vi "App - analyze RUS V6.vi"() -> ()   [LabVIEW 2015] (continued)
"last mod"=timestamp(3493785599 s since 1904-01-01), "file name str"="D:\\Data\\Ultrasound\\LSCO\\LSCO22__130814c\\5_Cooling_2nd_try\\September_2014\\091714\\72.10600K_500_2500_2.10000V_0.00000T_Sep17-2014__03-59-59_001_091714.bin", "mod time(min)"=58229759.983333334, "file format"=enum."binary", "power(V)"=2.1, "Magn Field(T) "=0.0}, {"temperature"=72.039, "temperature str"="72.03900", "file path"=path "D:/Data/Ultrasound/LSCO/LSCO22__130814c/5_Cooling_2nd_try/September_2014/091714/72.03900K_500_2500_2.10000V_0.00000T_Sep17-2014__04-01-18_001_091714.bin", "last mod"=timestamp(3493785678 s since 1904-01-01), "file name str"="D:\\Data\\Ultrasound\\LSCO\\LSCO22__130814c\\5_Cooling_2nd_try\\September_2014\\091714\\72.03900K_500_2500_2.10000V_0.00000T_Sep17-2014__04-01-18_001_091714.bin", "mod time(min)"=58229761.3, "file format"=enum."binary", "power(V)"=2.1, "Magn Field(T) "=0.0}, {"temperature"=71.974, "temperature str"="71.97400", "file path"=path "D:/Data/Ultrasound/LSCO/LSCO22__130814c/5_Cooling_2nd_try/September_2014/091714/71.97400K_500_2500_2.10000V_0.00000T_Sep17-2014__04-02-38_001_091714.bin", "last mod"=timestamp(3493785758 s since 1904-01-01), "file name str"="D:\\Data\\Ultrasound\\LSCO\\LSCO22__130814c\\5_Cooling_2nd_try\\September_2014\\091714\\71.97400K_500_2500_2.10000V_0.00000T_Sep17-2014__04-02-38_001_091714.bin", "mod time(min)"=58229762.63333333, "file format"=enum."binary", "power(V)"=2.1, "Magn Field(T) "=0.0}, {"temperature"=71.908, "temperature str"="71.90800", "file path"=path "D:/Data/Ultrasound/LSCO/LSCO22__130814c/5_Cooling_2nd_try/September_2014/091714/71.90800K_500_2500_2.10000V_0.00000T_Sep17-2014__04-03-57_001_091714.bin", "last mod"=timestamp(3493785837 s since 1904-01-01), "file name str"="D:\\Data\\Ultrasound\\LSCO\\LSCO22__130814c\\5_Cooling_2nd_try\\September_2014\\091714\\71.90800K_500_2500_2.10000V_0.00000T_Sep17-2014__04-03-57_001_091714.bin", "mod time(min)"=58229763.95, "file format"=enum."binary", "power(V)"=2.1, "Magn Field(T) "=0.0}, {"temperature"=71.842, "temperature str"="71.84200", "file path"=path "D:/Data/Ultrasound/LSCO/LSCO22__130814c/5_Cooling_2nd_try/September_2014/091714/71.84200K_500_2500_2.10000V_0.00000T_Sep17-2014__04-05-17_001_091714.bin", "last mod"=timestamp(3493785917 s since 1904-01-01), "file name str"="D:\\Data\\Ultrasound\\LSCO\\LSCO22__130814c\\5_Cooling_2nd_try\\September_2014\\091714\\71.84200K_500_2500_2.10000V_0.00000T_Sep17-2014__04-05-17_001_091714.bin", "mod time(min)"=58229765.28333333, "file format"=enum."binary", "power(V)"=2.1, "Magn Field(T) "=0.0}, {"temperature"=71.776, "temperature str"="71.77600", "file path"=path "D:/Data/Ultrasound/LSCO/LSCO22__130814c/5_Cooling_2nd_try/September_2014/091714/71.77600K_500_2500_2.10000V_0.00000T_Sep17-2014__04-06-36_001_091714.bin", "last mod"=timestamp(3493785996 s since 1904-01-01), "file name str"="D:\\Data\\Ultrasound\\LSCO\\LSCO22__130814c\\5_Cooling_2nd_try\\September_2014\\091714\\71.77600K_500_2500_2.10000V_0.00000T_Sep17-2014__04-06-36_001_091714.bin", "mod time(min)"=58229766.6, "file format"=enum."binary", "power(V)"=2.1, "Magn Field(T) "=0.0}, {"temperature"=71.708, "temperature str"="71.70800", "file path"=path "D:/Data/Ultrasound/LSCO/LSCO22__130814c/5_Cooling_2nd_try/September_2014/091714/71.70800K_500_2500_2.10000V_0.00000T_Sep17-2014__04-07-55_001_091714.bin", "last mod"=timestamp(3493786075 s since 1904-01-01), "file name str"="D:\\Data\\Ultrasound\\LSCO\\LSCO22__130814c\\5_Cooling_2nd_try\\September_2014\\091714\\71.70800K_500_2500_2.10000V_0.00000T_Sep17-2014__04-07-55_001_091714.bin", "mod time(min)"=58229767.916666664, "file format"=enum."binary", "power(V)"=2.1, "Magn Field(T) "=0.0}, {"temperature"=71.643, "temperature str"="71.64300", "file path"=path "D:/Data/Ultrasound/LSCO/LSCO22__130814c/5_Cooling_2nd_try/September_2014/091714/71.64300K_500_2500_2.10000V_0.00000T_Sep17-2014__04-09-15_001_091714.bin", "last mod"=timestamp(3493786155 s since 1904-01-01), "file name str"="D:\\Data\\Ultrasound\\LSCO\\LSCO22__130814c\\5_Cooling_2nd_try\\September_2014\\091714\\71.64300K_500_2500_2.10000V_0.00000T_Sep17-2014__04-09-15_001_091714.bin", "mod time(min)"=58229769.25, "file format"=enum."binary", "power(V)"=2.1, "Magn Field(T) "=0.0}, {"temperature"=71.578, "temperature str"="71.57800", "file path"=path "D:/Data/Ultrasound/LSCO/LSCO22__130814c/5_Cooling_2nd_try/September_2014/091714/71.57800K_500_2500_2.10000V_0.00000T_Sep17-2014__04-10-34_001_091714.bin", "last mod"=timestamp(3493786234 s since 1904-01-01), "file name str"="D:\\Data\\Ultrasound\\LSCO\\LSCO22__130814c\\5_Cooling_2nd_try\\September_2014\\091714\\71.57800K_500_2500_2.10000V_0.00000T_Sep17-2014__04-10-34_001_091714.bin", "mod time(min)"=58229770.56666667, "file format"=enum."binary", "power(V)"=2.1, "Magn Field(T) "=0.0}, {"temperature"=71.514, "temperature str"="71.51400", "file path"=path "D:/Data/Ultrasound/LSCO/LSCO22__130814c/5_Cooling_2nd_try/September_2014/091714/71.51400K_500_2500_2.10000V_0.00000T_Sep17-2014__04-11-54_001_091714.bin", "last mod"=timestamp(3493786314 s since 1904-01-01), "file name str"="D:\\Data\\Ultrasound\\LSCO\\LSCO22__130814c\\5_Cooling_2nd_try\\September_2014\\091714\\71.51400K_500_2500_2.10000V_0.00000T_Sep17-2014__04-11-54_001_091714.bin", "mod time(min)"=58229771.9, "file format"=enum."binary", "power(V)"=2.1, "Magn Field(T) "=0.0}, {"temperature"=71.446, "temperature str"="71.44600", "file path"=path "D:/Data/Ultrasound/LSCO/LSCO22__130814c/5_Cooling_2nd_try/September_2014/091714/71.44600K_500_2500_2.10000V_0.00000T_Sep17-2014__04-13-13_001_091714.bin", "last mod"=timestamp(3493786393 s since 1904-01-01), "file name str"="D:\\Data\\Ultrasound\\LSCO\\LSCO22__130814c\\5_Cooling_2nd_try\\September_2014\\091714\\71.44600K_500_2500_2.10000V_0.00000T_Sep17-2014__04-13-13_001_091714.bin", "mod time(min)"=58229773.21666667, "file format"=enum."binary", "power(V)"=2.1, "Magn Field(T) "=0.0}, {"temperature"=71.383, "temperature str"="71.38300", "file path"=path "D:/Data/Ultrasound/LSCO/LSCO22__130814c/5_Cooling_2nd_try/September_2014/091714/71.38300K_500_2500_2.10000V_0.00000T_Sep17-2014__04-14-32_001_091714.bin", "last mod"=timestamp(3493786472 s since 1904-01-01), "file name str"="D:\\Data\\Ultrasound\\LSCO\\LSCO22__130814c\\5_Cooling_2nd_try\\September_2014\\091714\\71.38300K_500_2500_2.10000V_0.00000T_Sep17-2014__04-14-32_001_091714.bin", "mod time(min)"=58229774.53333333, "file format"=enum."binary", "power(V)"=2.1, "Magn Field(T) "=0.0}, {"temperature"=71.316, "temperature str"="71.31600", "file path"=path "D:/Data/Ultrasound/LSCO/LSCO22__130814c/5_Cooling_2nd_try/September_2014/091714/71.31600K_500_2500_2.10000V_0.00000T_Sep17-2014__04-15-52_001_091714.bin", "last mod"=timestamp(3493786552 s since 1904-01-01), "file name str"="D:\\Data\\Ultrasound\\LSCO\\LSCO22__130814c\\5_Cooling_2nd_try\\September_2014\\091714\\71.31600K_500_2500_2.10000V_0.00000T_Sep17-2014__04-15-52_001_091714.bin", "mod time(min)"=58229775.86666667, "file format"=enum."binary", "power(V)"=2.1, "Magn Field(T) "=0.0}, {"temperature"=71.25, "temperature str"="71.25000", "file path"=path "D:/Data/Ultrasound/LSCO/LSCO22__130814c/5_Cooling_2nd_try/September_2014/091714/71.25000K_500_2500_2.10000V_0.00000T_Sep17-2014__04-17-11_001_091714.bin", "last mod"=timestamp(3493786631 s since 1904-01-01), "file name str"="D:\\Data\\Ultrasound\\LSCO\\LSCO22__130814c\\5_Cooling_2nd_try\\September_2014\\091714\\71.25000K_500_2500_2.10000V_0.00000T_Sep17-2014__04-17-11_001_091714.bin", "mod time(min)"=58229777.18333333, "file format"=enum."binary", "power(V)"=2.1, "Magn Field(T) "=0.0}, {"temperature"=71.184, "temperature str"="71.18400", "file path"=path "D:/Data/Ultrasound/LSCO/LSCO22__130814c/5_Cooling_2nd_try/September_2014/091714/71.18400K_500_2500_2.10000V_0.00000T_Sep17-2014__04-18-30_001_091714.bin", "last mod"=timestamp(3493786710 s since 1904-01-01), "file name str"="D:\\Data\\Ultrasound\\LSCO\\LSCO22__130814c\\5_Cooling_2nd_try\\September_2014\\091714\\71.18400K_500_2500_2.10000V_0.00000T_Sep17-2014__04-18-30_001_091714.bin", "mod time(min)"=58229778.5, "file format"=enum."binary", "power(V)"=2.1, "Magn Field(T) "=0.0}, {"temperature"=71.122, "temperature str"="71.12200", "file path"=path "D:/Data/Ultrasound/LSCO/LSCO22__130814c/5_Cooling_2nd_try/September_2014/091714/71.12200K_500_2500_2.10000V_0.00000T_Sep17-2014__04-19-50_001_091714.bin", "last mod"=timestamp(3493786790 s since 1904-01-01), "file name str"="D:\\Data\\Ultrasound\\LSCO\\LSCO22__130814c\\5_Cooling_2nd_try\\September_2014\\091714\\71.12200K_500_2500_2.10000V_0.00000T_Sep17-2014__04-19-50_001_091714.bin", "mod time(min)"=58229779.833333336, "file format"=enum."binary", "power(V)"=2.1, "Magn Field(T) "=0.0}, {"temperature"=71.056, "temperature str"="71.05600", "file path"=path "D:/Data/Ultrasound/LSCO/LSCO22__130814c/5_Cooling_2nd_try/September_2014/091714/71.05600K_500_2500_2.10000V_0.00000T_Sep17-2014__04-21-09_001_091714.bin", "last mod"=timestamp(3493786869 s since 1904-01-01), "file name str"="D:\\Data\\Ultrasound\\LSCO\\LSCO22__130814c\\5_Cooling_2nd_try\\September_2014\\091714\\71.05600K_500_2500_2.10000V_0.00000T_Sep17-2014__04-21-09_001_091714.bin", "mod time(min)"=58229781.15, "file format"=enum."binary", "power(V)"=2.1, "Magn Field(T) "=0.0}, {"temperature"=70.993, "temperature str"="70.99300", "file path"=path "D:/Data/Ultrasound/LSCO/LSCO22__130814c/5_Cooling_2nd_try/September_2014/091714/70.99300K_500_2500_2.10000V_0.00000T_Sep17-2014__04-22-29_001_091714.bin", "last mod"=timestamp(3493786949 s since 1904-01-01), "file name str"="D:\\Data\\Ultrasound\\LSCO\\LSCO22__130814c\\5_Cooling_2nd_try\\September_2014\\091714\\70.99300K_500_2500_2.10000V_0.00000T_Sep17-2014__04-22-29_001_091714.bin", "mod time(min)"=58229782.483333334, "file format"=enum."binary", "power(V)"=2.1, "Magn Field(T) "=0.0}, {"temperature"=70.928, "temperature str"="70.92800", "file path"=path "D:/Data/Ultrasound/LSCO/LSCO22__130814c/5_Cooling_2nd_try/September_2014/091714/70.92800K_500_2500_2.10000V_0.00000T_Sep17-2014__04-23-48_001_091714.bin", "last mod"=timestamp(3493787028 s since 1904-01-01), "file name str"="D:\\Data\\Ultrasound\\LSCO\\LSCO22__130814c\\5_Cooling_2nd_try\\September_2014\\091714\\70.92800K_500_2500_2.10000V_0.00000T_Sep17-2014__04-23-48_001_091714.bin", "mod time(min)"=58229783.8, "file format"=enum."binary", "power(V)"=2.1, "Magn Field(T) "=0.0}, {"temperature"=70.86, "temperature str"="70.86000", "file path"=path "D:/Data/Ultrasound/LSCO/LSCO22__130814c/5_Cooling_2nd_try/September_2014/091714/70.86000K_500_2500_2.10000V_0.00000T_Sep17-2014__04-25-07_001_091714.bin", "last mod"=timestamp(3493787107 s since 1904-01-01), "file name str"="D:\\Data\\Ultrasound\\LSCO\\LSCO22__130814c\\5_Cooling_2nd_try\\September_2014\\091714\\70.86000K_500_2500_2.10000V_0.00000T_Sep17-2014__04-25-07_001_091714.bin", "mod time(min)"=58229785.11666667, "file format"=enum."binary", "power(V)"=2.1, "Magn Field(T) "=0.0}, {"temperature"=70.8, "temperature str"="70.80000", "file path"=path "D:/Data/Ultrasound/LSCO/LSCO22__130814c/5_Cooling_2nd_try/September_2014/091714/70.80000K_500_2500_2.10000V_0.00000T_Sep17-2014__04-26-27_001_091714.bin", "last mod"=timestamp(3493787187 s since 1904-01-01), "file name str"="D:\\Data\\Ultrasound\\LSCO\\LSCO22__130814c\\5_Cooling_2nd_try\\September_2014\\091714\\70.80000K_500_2500_2.10000V_0.00000T_Sep17-2014__04-26-27_001_091714.bin", "mod time(min)"=58229786.45, "file format"=enum."binary", "power(V)"=2.1, "Magn Field(T) "=0.0}, {"temperature"=70.734, "temperature str"="70.73400", "file path"=path "D:/Data/Ultrasound/LSCO/LSCO22__130814c/5_Cooling_2nd_try/September_2014/091714/70.73400K_500_2500_2.10000V_0.00000T_Sep17-2014__04-27-46_001_091714.bin", "last mod"=timestamp(3493787266 s since 1904-01-01), "file name str"="D:\\Data\\Ultrasound\\LSCO\\LSCO22__130814c\\5_Cooling_2nd_try\\September_2014\\091714\\70.73400K_500_2500_2.10000V_0.00000T_Sep17-2014__04-27-46_001_091714.bin", "mod time(min)"=58229787.766666666, "file format"=enum."binary", "power(V)"=2.1, "Magn Field(T) "=0.0}, {"temperature"=70.67, "temperature str"="70.67000", "file path"=path "D:/Data/Ultrasound/LSCO/LSCO22__130814c/5_Cooling_2nd_try/September_2014/091714/70.67000K_500_2500_2.10000V_0.00000T_Sep17-2014__04-29-06_001_091714.bin", "last mod"=timestamp(3493787346 s since 1904-01-01), "file name str"="D:\\Data\\Ultrasound\\LSCO\\LSCO22__130814c\\5_Cooling_2nd_try\\September_2014\\091714\\70.67000K_500_2500_2.10000V_0.00000T_Sep17-2014__04-29-06_001_091714.bin", "mod time(min)"=58229789.1, "file format"=enum."binary", "power(V)"=2.1, "Magn Field(T) "=0.0}, {"temperature"=70.607, "temperature str"="70.60700", "file path"=path "D:/Data/Ultrasound/LSCO/LSCO22__130814c/5_Cooling_2nd_try/September_2014/091714/70.60700K_500_2500_2.10000V_0.00000T_Sep17-2014__04-30-25_001_091714.bin", "last mod"=timestamp(3493787425 s since 1904-01-01), "file name str"="D:\\Data\\Ultrasound\\LSCO\\LSCO22__130814c\\5_Cooling_2nd_try\\September_2014\\091714\\70.60700K_500_2500_2.10000V_0.00000T_Sep17-2014__04-30-25_001_091714.bin", "mod time(min)"=58229790.416666664, "file format"=enum."binary", "power(V)"=2.1, "Magn Field(T) "=0.0}, {"temperature"=70.54, "temperature str"="70.54000", "file path"=path "D:/Data/Ultrasound/LSCO/LSCO22__130814c/5_Cooling_2nd_try/September_2014/091714/70.54000K_500_2500_2.10000V_0.00000T_Sep17-2014__04-31-44_001_091714.bin", "last mod"=timestamp(3493787504 s since 1904-01-01), "file name str"="D:\\Data\\Ultrasound\\LSCO\\LSCO22__130814c\\5_Cooling_2nd_try\\September_2014\\091714\\70.54000K_500_2500_2.10000V_0.00000T_Sep17-2014__04-31-44_001_091714.bin", "mod time(min)"=58229791.733333334, "file format"=enum."binary", "power(V)"=2.1, "Magn Field(T) "=0.0}, {"temperature"=70.48, "temperature str"="70.48000", "file path"=path "D:/Data/Ultrasound/LSCO/LSCO22__130814c/5_Cooling_2nd_try/September_2014/091714/70.48000K_500_2500_2.10000V_0.00000T_Sep17-2014__04-33-04_001_091714.bin", "last mod"=timestamp(3493787584 s since 1904-01-01), "file name str"="D:\\Data\\Ultrasound\\LSCO\\LSCO22__130814c\\5_Cooling_2nd_try\\September_2014\\091714\\70.48000K_500_2500_2.10000V_0.00000T_Sep17-2014__04-33-04_001_091714.bin", "mod time(min)"=58229793.06666667, "file format"=enum."binary", "power(V)"=2.1, "Magn Field(T) "=0.0}, {"temperature"=70.414, "temperature str"="70.41400", "file path"=path "D:/Data/Ultrasound/LSCO/LSCO22__130814c/5_Cooling_2nd_try/September_2014/091714/70.41400K_500_2500_2.10000V_0.00000T_Sep17-2014__04-34-23_001_091714.bin", "last mod"=timestamp(3493787663 s since 1904-01-01), "file name str"="D:\\Data\\Ultrasound\\LSCO\\LSCO22__130814c\\5_Cooling_2nd_try\\September_2014\\091714\\70.41400K_500_2500_2.10000V_0.00000T_Sep17-2014__04-34-23_001_091714.bin", "mod time(min)"=58229794.38333333, "file format"=enum."binary", "power(V)"=2.1, "Magn Field(T) "=0.0}, {"temperature"=70.35, "temperature str"="70.35000", "file path"=path "D:/Data/Ultrasound/LSCO/LSCO22__130814c/5_Cooling_2nd_try/September_2014/091714/70.35000K_500_2500_2.10000V_0.00000T_Sep17-2014__04-35-42_001_091714.bin", "last mod"=timestamp(3493787742 s since 1904-01-01), "file name str"="D:\\Data\\Ultrasound\\LSCO\\LSCO22__130814c\\5_Cooling_2nd_try\\September_2014\\091714\\70.35000K_500_2500_2.10000V_0.00000T_Sep17-2014__04-35-42_001_091714.bin", "mod time(min)"=58229795.7, "file format"=enum."binary", "power(V)"=2.1, "Magn Field(T) "=0.0}, {"temperature"=70.285, "temperature str"="70.28500", "file path"=path "D:/Data/Ultrasound/LSCO/LSCO22__130814c/5_Cooling_2nd_try/September_2014/091714/70.28500K_500_2500_2.10000V_0.00000T_Sep17-2014__04-37-02_001_091714.bin", "last mod"=timestamp(3493787822 s since 1904-01-01), "file name str"="D:\\Data\\Ultrasound\\LSCO\\LSCO22__130814c\\5_Cooling_2nd_try\\September_2014\\091714\\70.28500K_500_2500_2.10000V_0.00000T_Sep17-2014__04-37-02_001_091714.bin", "mod time(min)"=58229797.03333333, "file format"=enum."binary", "power(V)"=2.1, "Magn Field(T) "=0.0}, {"temperature"=70.221, "temperature str"="70.22100", "file path"=path "D:/Data/Ultrasound/LSCO/LSCO22__130814c/5_Cooling_2nd_try/September_2014/091714/70.22100K_500_2500_2.10000V_0.00000T_Sep17-2014__04-38-21_001_091714.bin", "last mod"=timestamp(3493787901 s since 1904-01-01), "file name str"="D:\\Data\\Ultrasound\\LSCO\\LSCO22__130814c\\5_Cooling_2nd_try\\September_2014\\091714\\70.22100K_500_2500_2.10000V_0.00000T_Sep17-2014__04-38-21_001_091714.bin", "mod time(min)"=58229798.35, "file format"=enum."binary", "power(V)"=2.1, "Magn Field(T) "=0.0}, {"temperature"=70.16, "temperature str"="70.16000", "file path"=path "D:/Data/Ultrasound/LSCO/LSCO22__130814c/5_Cooling_2nd_try/September_2014/091714/70.16000K_500_2500_2.10000V_0.00000T_Sep17-2014__04-39-41_001_091714.bin", "last mod"=timestamp(3493787981 s since 1904-01-01), "file name str"="D:\\Data\\Ultrasound\\LSCO\\LSCO22__130814c\\5_Cooling_2nd_try\\September_2014\\091714\\70.16000K_500_2500_2.10000V_0.00000T_Sep17-2014__04-39-41_001_091714.bin", "mod time(min)"=58229799.68333333, "file format"=enum."binary", "power(V)"=2.1, "Magn Field(T) "=0.0}, {"temperature"=70.095, "temperature str"="70.09500", "file path"=path "D:/Data/Ultrasound/LSCO/LSCO22__130814c/5_Cooling_2nd_try/September_2014/091714/70.09500K_500_2500_2.10000V_0.00000T_Sep17-2014__04-41-00_001_091714.bin", "last mod"=timestamp(3493788060 s since 1904-01-01), "file name str"="D:\\Data\\Ultrasound\\LSCO\\LSCO22__130814c\\5_Cooling_2nd_try\\September_2014\\091714\\70.09500K_500_2500_2.10000V_0.00000T_Sep17-2014__04-41-00_001_091714.bin", "mod time(min)"=58229801.0, "file format"=enum."binary", "power(V)"=2.1, "Magn Field(T) "=0.0}, {"temperature"=70.033, "temperature str"="70.03300", "file path"=path "D:/Data/Ultrasound/LSCO/LSCO22__130814c/5_Cooling_2nd_try/September_2014/091714/70.03300K_500_2500_2.10000V_0.00000T_Sep17-2014__04-42-19_001_091714.bin", "last mod"=timestamp(3493788139 s since 1904-01-01), "file name str"="D:\\Data\\Ultrasound\\LSCO\\LSCO22__130814c\\5_Cooling_2nd_try\\September_2014\\091714\\70.03300K_500_2500_2.10000V_0.00000T_Sep17-2014__04-42-19_001_091714.bin", "mod time(min)"=58229802.31666667, "file format"=enum."binary", "power(V)"=2.1, "Magn Field(T) "=0.0}, {"temperature"=69.969, "temperature str"="69.96900", "file path"=path "D:/Data/Ultrasound/LSCO/LSCO22__130814c/5_Cooling_2nd_try/September_2014/091714/69.96900K_500_2500_2.10000V_0.00000T_Sep17-2014__04-43-39_001_091714.bin", "last mod"=timestamp(3493788219 s since 1904-01-01), "file name str"="D:\\Data\\Ultrasound\\LSCO\\LSCO22__130814c\\5_Cooling_2nd_try\\September_2014\\091714\\69.96900K_500_2500_2.10000V_0.00000T_Sep17-2014__04-43-39_001_091714.bin", "mod time(min)"=58229803.65, "file format"=enum."binary", "power(V)"=2.1, "Magn Field(T) "=0.0}, {"temperature"=69.905, "temperature str"="69.90500", "file path"=path "D:/Data/Ultrasound/LSCO/LSCO22__130814c/5_Cooling_2nd_try/September_2014/091714/69.90500K_500_2500_2.10000V_0.00000T_Sep17-2014__04-44-58_001_091714.bin", "last mod"=timestamp(3493788298 s since 1904-01-01), "file name str"="D:\\Data\\Ultrasound\\LSCO\\LSCO22__130814c\\5_Cooling_2nd_try\\September_2014\\091714\\69.90500K_500_2500_2.10000V_0.00000T_Sep17-2014__04-44-58_001_091714.bin", "mod time(min)"=58229804.96666667, "file format"=enum."binary", "power(V)"=2.1, "Magn Field(T) "=0.0}, {"temperature"=69.845, "temperature str"="69.84500", "file path"=path "D:/Data/Ultrasound/LSCO/LSCO22__130814c/5_Cooling_2nd_try/September_2014/091714/69.84500K_500_2500_2.10000V_0.00000T_Sep17-2014__04-46-18_001_091714.bin", "last mod"=timestamp(3493788378 s since 1904-01-01), "file name str"="D:\\Data\\Ultrasound\\LSCO\\LSCO22__130814c\\5_Cooling_2nd_try\\September_2014\\091714\\69.84500K_500_2500_2.10000V_0.00000T_Sep17-2014__04-46-18_001_091714.bin", "mod time(min)"=58229806.3, "file format"=enum."binary", "power(V)"=2.1, "Magn Field(T) "=0.0}, {"temperature"=69.78, "temperature str"="69.78000", "file path"=path "D:/Data/Ultrasound/LSCO/LSCO22__130814c/5_Cooling_2nd_try/September_2014/091714/69.78000K_500_2500_2.10000V_0.00000T_Sep17-2014__04-47-37_001_091714.bin", "last mod"=timestamp(3493788457 s since 1904-01-01), "file name str"="D:\\Data\\Ultrasound\\LSCO\\LSCO22__130814c\\5_Cooling_2nd_try\\September_2014\\091714\\69.78000K_500_2500_2.10000V_0.00000T_Sep17-2014__04-47-37_001_091714.bin", "mod time(min)"=58229807.61666667, "file format"=enum."binary", "power(V)"=2.1, "Magn Field(T) "=0.0}, {"temperature"=69.717, "temperature str"="69.71700", "file path"=path "D:/Data/Ultrasound/LSCO/LSCO22__130814c/5_Cooling_2nd_try/September_2014/091714/69.71700K_500_2500_2.10000V_0.00000T_Sep17-2014__04-48-56_001_091714.bin", "last mod"=timestamp(3493788536 s since 1904-01-01), "file name str"="D:\\Data\\Ultrasound\\LSCO\\LSCO22__130814c\\5_Cooling_2nd_try\\September_2014\\091714\\69.71700K_500_2500_2.10000V_0.00000T_Sep17-2014__04-48-56_001_091714.bin", "mod time(min)"=58229808.93333333, "file format"=enum."binary", "power(V)"=2.1, "Magn Field(T) "=0.0}, {"temperature"=69.656, "temperature str"="69.65600", "file path"=path "D:/Data/Ultrasound/LSCO/LSCO22__130814c/5_Cooling_2nd_try/September_2014/091714/69.65600K_500_2500_2.10000V_0.00000T_Sep17-2014__04-50-16_001_091714.bin", "last mod"=timestamp(3493788616 s since 1904-01-01), "file name str"="D:\\Data\\Ultrasound\\LSCO\\LSCO22__130814c\\5_Cooling_2nd_try\\September_2014\\091714\\69.65600K_500_2500_2.10000V_0.00000T_Sep17-2014__04-50-16_001_091714.bin", "mod time(min)"=58229810.266666666, "file format"=enum."binary", "power(V)"=2.1, "Magn Field(T) "=0.0}, {"temperature"=69.592, "temperature str"="69.59200", "file path"=path "D:/Data/Ultrasound/LSCO/LSCO22__130814c/5_Cooling_2nd_try/September_2014/091714/69.59200K_500_2500_2.10000V_0.00000T_Sep17-2014__04-51-35_001_091714.bin", "last mod"=timestamp(3493788695 s since 1904-01-01), "file name str"="D:\\Data\\Ultrasound\\LSCO\\LSCO22__130814c\\5_Cooling_2nd_try\\September_2014\\091714\\69.59200K_500_2500_2.10000V_0.00000T_Sep17-2014__04-51-35_001_091714.bin", "mod time(min)"=58229811.583333336, "file format"=enum."binary", "power(V)"=2.1, "Magn Field(T) "=0.0}, {"temperature"=69.531, "temperature str"="69.53100", "file path"=path "D:/Data/Ultrasound/LSCO/LSCO22__130814c/5_Cooling_2nd_try/September_2014/091714/69.53100K_500_2500_2.10000V_0.00000T_Sep17-2014__04-52-54_001_091714.bin", "last mod"=timestamp(3493788774 s since 1904-01-01), "file name str"="D:\\Data\\Ultrasound\\LSCO\\LSCO22__130814c\\5_Cooling_2nd_try\\September_2014\\091714\\69.53100K_500_2500_2.10000V_0.00000T_Sep17-2014__04-52-54_001_091714.bin", "mod time(min)"=58229812.9, "file format"=enum."binary", "power(V)"=2.1, "Magn Field(T) "=0.0}, {"temperature"=69.468, "temperature str"="69.46800", "file path"=path "D:/Data/Ultrasound/LSCO/LSCO22__130814c/5_Cooling_2nd_try/September_2014/091714/69.46800K_500_2500_2.10000V_0.00000T_Sep17-2014__04-54-14_001_091714.bin", "last mod"=timestamp(3493788854 s since 1904-01-01), "file name str"="D:\\Data\\Ultrasound\\LSCO\\LSCO22__130814c\\5_Cooling_2nd_try\\September_2014\\091714\\69.46800K_500_2500_2.10000V_0.00000T_Sep17-2014__04-54-14_001_091714.bin", "mod time(min)"=58229814.233333334, "file format"=enum."binary", "power(V)"=2.1, "Magn Field(T) "=0.0}, {"temperature"=69.402, "temperature str"="69.40200", "file path"=path "D:/Data/Ultrasound/LSCO/LSCO22__130814c/5_Cooling_2nd_try/September_2014/091714/69.40200K_500_2500_2.10000V_0.00000T_Sep17-2014__04-55-33_001_091714.bin", "last mod"=timestamp(3493788933 s since 1904-01-01), "file name str"="D:\\Data\\Ultrasound\\LSCO\\LSCO22__130814c\\5_Cooling_2nd_try\\September_2014\\091714\\69.40200K_500_2500_2.10000V_0.00000T_Sep17-2014__04-55-33_001_091714.bin", "mod time(min)"=58229815.55, "file format"=enum."binary", "power(V)"=2.1, "Magn Field(T) "=0.0}, {"temperature"=69.343, "temperature str"="69.34300", "file path"=path "D:/Data/Ultrasound/LSCO/LSCO22__130814c/5_Cooling_2nd_try/September_2014/091714/69.34300K_500_2500_2.10000V_0.00000T_Sep17-2014__04-56-53_001_091714.bin", "last mod"=timestamp(3493789013 s since 1904-01-01), "file name str"="D:\\Data\\Ultrasound\\LSCO\\LSCO22__130814c\\5_Cooling_2nd_try\\September_2014\\091714\\69.34300K_500_2500_2.10000V_0.00000T_Sep17-2014__04-56-53_001_091714.bin", "mod time(min)"=58229816.88333333, "file format"=enum."binary", "power(V)"=2.1, "Magn Field(T) "=0.0}, {"temperature"=69.279, "temperature str"="69.27900", "file path"=path "D:/Data/Ultrasound/LSCO/LSCO22__130814c/5_Cooling_2nd_try/September_2014/091714/69.27900K_500_2500_2.10000V_0.00000T_Sep17-2014__04-58-12_001_091714.bin", "last mod"=timestamp(3493789092 s since 1904-01-01), "file name str"="D:\\Data\\Ultrasound\\LSCO\\LSCO22__130814c\\5_Cooling_2nd_try\\September_2014\\091714\\69.27900K_500_2500_2.10000V_0.00000T_Sep17-2014__04-58-12_001_091714.bin", "mod time(min)"=58229818.2, "file format"=enum."binary", "power(V)"=2.1, "Magn Field(T) "=0.0}, {"temperature"=69.219, "temperature str"="69.21900", "file path"=path "D:/Data/Ultrasound/LSCO/LSCO22__130814c/5_Cooling_2nd_try/September_2014/091714/69.21900K_500_2500_2.10000V_0.00000T_Sep17-2014__04-59-31_001_091714.bin", "last mod"=timestamp(3493789171 s since 1904-01-01), "file name str"="D:\\Data\\Ultrasound\\LSCO\\LSCO22__130814c\\5_Cooling_2nd_try\\September_2014\\091714\\69.21900K_500_2500_2.10000V_0.00000T_Sep17-2014__04-59-31_001_091714.bin", "mod time(min)"=58229819.516666666, "file format"=enum."binary", "power(V)"=2.1, "Magn Field(T) "=0.0}, {"temperature"=69.155, "temperature str"="69.15500", "file path"=path "D:/Data/Ultrasound/LSCO/LSCO22__130814c/5_Cooling_2nd_try/September_2014/091714/69.15500K_500_2500_2.10000V_0.00000T_Sep17-2014__05-00-51_001_091714.bin", "last mod"=timestamp(3493789251 s since 1904-01-01), "file name str"="D:\\Data\\Ultrasound\\LSCO\\LSCO22__130814c\\5_Cooling_2nd_try\\September_2014\\091714\\69.15500K_500_2500_2.10000V_0.00000T_Sep17-2014__05-00-51_001_091714.bin", "mod time(min)"=58229820.85, "file format"=enum."binary", "power(V)"=2.1, "Magn Field(T) "=0.0}, {"temperature"=69.092, "temperature str"="69.09200", "file path"=path "D:/Data/Ultrasound/LSCO/LSCO22__130814c/5_Cooling_2nd_try/September_2014/091714/69.09200K_500_2500_2.10000V_0.00000T_Sep17-2014__05-02-10_001_091714.bin", "last mod"=timestamp(3493789330 s since 1904-01-01), "file name str"="D:\\Data\\Ultrasound\\LSCO\\LSCO22__130814c\\5_Cooling_2nd_try\\September_2014\\091714\\69.09200K_500_2500_2.10000V_0.00000T_Sep17-2014__05-02-10_001_091714.bin", "mod time(min)"=58229822.166666664, "file format"=enum."binary", "power(V)"=2.1, "Magn Field(T) "=0.0}, {"temperature"=69.033, "temperature str"="69.03300", "file path"=path "D:/Data/Ultrasound/LSCO/LSCO22__130814c/5_Cooling_2nd_try/September_2014/091714/69.03300K_500_2500_2.10000V_0.00000T_Sep17-2014__05-03-30_001_091714.bin", "last mod"=timestamp(3493789410 s since 1904-01-01), "file name str"="D:\\Data\\Ultrasound\\LSCO\\LSCO22__130814c\\5_Cooling_2nd_try\\September_2014\\091714\\69.03300K_500_2500_2.10000V_0.00000T_Sep17-2014__05-03-30_001_091714.bin", "mod time(min)"=58229823.5, "file format"=enum."binary", "power(V)"=2.1, "Magn Field(T) "=0.0}, {"temperature"=68.969, "temperature str"="68.96900", "file path"=path "D:/Data/Ultrasound/LSCO/LSCO22__130814c/5_Cooling_2nd_try/September_2014/091714/68.96900K_500_2500_2.10000V_0.00000T_Sep17-2014__05-04-49_001_091714.bin", "last mod"=timestamp(3493789489 s since 1904-01-01), "file name str"="D:\\Data\\Ultrasound\\LSCO\\LSCO22__130814c\\5_Cooling_2nd_try\\September_2014\\091714\\68.96900K_500_2500_2.10000V_0.00000T_Sep17-2014__05-04-49_001_091714.bin", "mod time(min)"=58229824.81666667, "file format"=enum."binary", "power(V)"=2.1, "Magn Field(T) "=0.0}, {"temperature"=68.909, "temperature str"="68.90900", "file path"=path "D:/Data/Ultrasound/LSCO/LSCO22__130814c/5_Cooling_2nd_try/September_2014/091714/68.90900K_500_2500_2.10000V_0.00000T_Sep17-2014__05-06-08_001_091714.bin", "last mod"=timestamp(3493789568 s since 1904-01-01), "file name str"="D:\\Data\\Ultrasound\\LSCO\\LSCO22__130814c\\5_Cooling_2nd_try\\September_2014\\091714\\68.90900K_500_2500_2.10000V_0.00000T_Sep17-2014__05-06-08_001_091714.bin", "mod time(min)"=58229826.13333333, "file format"=enum."binary", "power(V)"=2.1, "Magn Field(T) "=0.0}, {"temperature"=68.845, "temperature str"="68.84500", "file path"=path "D:/Data/Ultrasound/LSCO/LSCO22__130814c/5_Cooling_2nd_try/September_2014/091714/68.84500K_500_2500_2.10000V_0.00000T_Sep17-2014__05-07-28_001_091714.bin", "last mod"=timestamp(3493789648 s since 1904-01-01), "file name str"="D:\\Data\\Ultrasound\\LSCO\\LSCO22__130814c\\5_Cooling_2nd_try\\September_2014\\091714\\68.84500K_500_2500_2.10000V_0.00000T_Sep17-2014__05-07-28_001_091714.bin", "mod time(min)"=58229827.46666667, "file format"=enum."binary", "power(V)"=2.1, "Magn Field(T) "=0.0}, {"temperature"=68.784, "temperature str"="68.78400", "file path"=path "D:/Data/Ultrasound/LSCO/LSCO22__130814c/5_Cooling_2nd_try/September_2014/091714/68.78400K_500_2500_2.10000V_0.00000T_Sep17-2014__05-08-47_001_091714.bin", "last mod"=timestamp(3493789727 s since 1904-01-01), "file name str"="D:\\Data\\Ultrasound\\LSCO\\LSCO22__130814c\\5_Cooling_2nd_try\\September_2014\\091714\\68.78400K_500_2500_2.10000V_0.00000T_Sep17-2014__05-08-47_001_091714.bin", "mod time(min)"=58229828.78333333, "file format"=enum."binary", "power(V)"=2.1, "Magn Field(T) "=0.0}, {"temperature"=68.723, "temperature str"="68.72300", "file path"=path "D:/Data/Ultrasound/LSCO/LSCO22__130814c/5_Cooling_2nd_try/September_2014/091714/68.72300K_500_2500_2.10000V_0.00000T_Sep17-2014__05-10-06_001_091714.bin", "last mod"=timestamp(3493789806 s since 1904-01-01), "file name str"="D:\\Data\\Ultrasound\\LSCO\\LSCO22__130814c\\5_Cooling_2nd_try\\September_2014\\091714\\68.72300K_500_2500_2.10000V_0.00000T_Sep17-2014__05-10-06_001_091714.bin", "mod time(min)"=58229830.1, "file format"=enum."binary", "power(V)"=2.1, "Magn Field(T) "=0.0}, {"temperature"=68.661, "temperature str"="68.66100", "file path"=path "D:/Data/Ultrasound/LSCO/LSCO22__130814c/5_Cooling_2nd_try/September_2014/091714/68.66100K_500_2500_2.10000V_0.00000T_Sep17-2014__05-11-26_001_091714.bin", "last mod"=timestamp(3493789886 s since 1904-01-01), "file name str"="D:\\Data\\Ultrasound\\LSCO\\LSCO22__130814c\\5_Cooling_2nd_try\\September_2014\\091714\\68.66100K_500_2500_2.10000V_0.00000T_Sep17-2014__05-11-26_001_091714.bin", "mod time(min)"=58229831.43333333, "file format"=enum."binary", "power(V)"=2.1, "Magn Field(T) "=0.0}, {"temperature"=68.599, "temperature str"="68.59900", "file path"=path "D:/Data/Ultrasound/LSCO/LSCO22__130814c/5_Cooling_2nd_try/September_2014/091714/68.59900K_500_2500_2.10000V_0.00000T_Sep17-2014__05-12-45_001_091714.bin", "last mod"=timestamp(3493789965 s since 1904-01-01), "file name str"="D:\\Data\\Ultrasound\\LSCO\\LSCO22__130814c\\5_Cooling_2nd_try\\September_2014\\091714\\68.59900K_500_2500_2.10000V_0.00000T_Sep17-2014__05-12-45_001_091714.bin", "mod time(min)"=58229832.75, "file format"=enum."binary", "power(V)"=2.1, "Magn Field(T) "=0.0}, {"temperature"=68.538, "temperature str"="68.53800", "file path"=path "D:/Data/Ultrasound/LSCO/LSCO22__130814c/5_Cooling_2nd_try/September_2014/091714/68.53800K_500_2500_2.10000V_0.00000T_Sep17-2014__05-14-05_001_091714.bin", "last mod"=timestamp(3493790045 s since 1904-01-01), "file name str"="D:\\Data\\Ultrasound\\LSCO\\LSCO22__130814c\\5_Cooling_2nd_try\\September_2014\\091714\\68.53800K_500_2500_2.10000V_0.00000T_Sep17-2014__05-14-05_001_091714.bin", "mod time(min)"=58229834.083333336, "file format"=enum."binary", "power(V)"=2.1, "Magn Field(T) "=0.0}, {"temperature"=68.475, "temperature str"="68.47500", "file path"=path "D:/Data/Ultrasound/LSCO/LSCO22__130814c/5_Cooling_2nd_try/September_2014/091714/68.47500K_500_2500_2.10000V_0.00000T_Sep17-2014__05-15-24_001_091714.bin", "last mod"=timestamp(3493790124 s since 1904-01-01), "file name str"="D:\\Data\\Ultrasound\\LSCO\\LSCO22__130814c\\5_Cooling_2nd_try\\September_2014\\091714\\68.47500K_500_2500_2.10000V_0.00000T_Sep17-2014__05-15-24_001_091714.bin", "mod time(min)"=58229835.4, "file format"=enum."binary", "power(V)"=2.1, "Magn Field(T) "=0.0}, {"temperature"=68.415, "temperature str"="68.41500", "file path"=path "D:/Data/Ultrasound/LSCO/LSCO22__130814c/5_Cooling_2nd_try/September_2014/091714/68.41500K_500_2500_2.10000V_0.00000T_Sep17-2014__05-16-43_001_091714.bin", "last mod"=timestamp(3493790203 s since 1904-01-01), "file name str"="D:\\Data\\Ultrasound\\LSCO\\LSCO22__130814c\\5_Cooling_2nd_try\\September_2014\\091714\\68.41500K_500_2500_2.10000V_0.00000T_Sep17-2014__05-16-43_001_091714.bin", "mod time(min)"=58229836.71666667, "file format"=enum."binary", "power(V)"=2.1, "Magn Field(T) "=0.0}, {"temperature"=68.353, "temperature str"="68.35300", "file path"=path "D:/Data/Ultrasound/LSCO/LSCO22__130814c/5_Cooling_2nd_try/September_2014/091714/68.35300K_500_2500_2.10000V_0.00000T_Sep17-2014__05-18-03_001_091714.bin", "last mod"=timestamp(3493790283 s since 1904-01-01), "file name str"="D:\\Data\\Ultrasound\\LSCO\\LSCO22__130814c\\5_Cooling_2nd_try\\September_2014\\091714\\68.35300K_500_2500_2.10000V_0.00000T_Sep17-2014__05-18-03_001_091714.bin", "mod time(min)"=58229838.05, "file format"=enum."binary", "power(V)"=2.1, "Magn Field(T) "=0.0}, {"temperature"=68.294, "temperature str"="68.29400", "file path"=path "D:/Data/Ultrasound/LSCO/LSCO22__130814c/5_Cooling_2nd_try/September_2014/091714/68.29400K_500_2500_2.10000V_0.00000T_Sep17-2014__05-19-22_001_091714.bin", "last mod"=timestamp(3493790362 s since 1904-01-01), "file name str"="D:\\Data\\Ultrasound\\LSCO\\LSCO22__130814c\\5_Cooling_2nd_try\\September_2014\\091714\\68.29400K_500_2500_2.10000V_0.00000T_Sep17-2014__05-19-22_001_091714.bin", "mod time(min)"=58229839.36666667, "file format"=enum."binary", "power(V)"=2.1, "Magn Field(T) "=0.0}, {"temperature"=68.232, "temperature str"="68.23200", "file path"=path "D:/Data/Ultrasound/LSCO/LSCO22__130814c/5_Cooling_2nd_try/September_2014/091714/68.23200K_500_2500_2.10000V_0.00000T_Sep17-2014__05-20-42_001_091714.bin", "last mod"=timestamp(3493790442 s since 1904-01-01), "file name str"="D:\\Data\\Ultrasound\\LSCO\\LSCO22__130814c\\5_Cooling_2nd_try\\September_2014\\091714\\68.23200K_500_2500_2.10000V_0.00000T_Sep17-2014__05-20-42_001_091714.bin", "mod time(min)"=58229840.7, "file format"=enum."binary", "power(V)"=2.1, "Magn Field(T) "=0.0}, {"temperature"=68.168, "temperature str"="68.16800", "file path"=path "D:/Data/Ultrasound/LSCO/LSCO22__130814c/5_Cooling_2nd_try/September_2014/091714/68.16800K_500_2500_2.10000V_0.00000T_Sep17-2014__05-22-01_001_091714.bin", "last mod"=timestamp(3493790521 s since 1904-01-01), "file name str"="D:\\Data\\Ultrasound\\LSCO\\LSCO22__130814c\\5_Cooling_2nd_try\\September_2014\\091714\\68.16800K_500_2500_2.10000V_0.00000T_Sep17-2014__05-22-01_001_091714.bin", "mod time(min)"=58229842.016666666, "file format"=enum."binary", "power(V)"=2.1, "Magn Field(T) "=0.0}, {"temperature"=68.111, "temperature str"="68.11100", "file path"=path "D:/Data/Ultrasound/LSCO/LSCO22__130814c/5_Cooling_2nd_try/September_2014/091714/68.11100K_500_2500_2.10000V_0.00000T_Sep17-2014__05-23-20_001_091714.bin", "last mod"=timestamp(3493790600 s since 1904-01-01), "file name str"="D:\\Data\\Ultrasound\\LSCO\\LSCO22__130814c\\5_Cooling_2nd_try\\September_2014\\091714\\68.11100K_500_2500_2.10000V_0.00000T_Sep17-2014__05-23-20_001_091714.bin", "mod time(min)"=58229843.333333336, "file format"=enum."binary", "power(V)"=2.1, "Magn Field(T) "=0.0}, {"temperature"=68.048, "temperature str"="68.04800", "file path"=path "D:/Data/Ultrasound/LSCO/LSCO22__130814c/5_Cooling_2nd_try/September_2014/091714/68.04800K_500_2500_2.10000V_0.00000T_Sep17-2014__05-24-40_001_091714.bin", "last mod"=timestamp(3493790680 s since 1904-01-01), "file name str"="D:\\Data\\Ultrasound\\LSCO\\LSCO22__130814c\\5_Cooling_2nd_try\\September_2014\\091714\\68.04800K_500_2500_2.10000V_0.00000T_Sep17-2014__05-24-40_001_091714.bin", "mod time(min)"=58229844.666666664, "file format"=enum."binary", "power(V)"=2.1, "Magn Field(T) "=0.0}, {"temperature"=67.989, "temperature str"="67.98900", "file path"=path "D:/Data/Ultrasound/LSCO/LSCO22__130814c/5_Cooling_2nd_try/September_2014/091714/67.98900K_500_2500_2.10000V_0.00000T_Sep17-2014__05-25-59_001_091714.bin", "last mod"=timestamp(3493790759 s since 1904-01-01), "file name str"="D:\\Data\\Ultrasound\\LSCO\\LSCO22__130814c\\5_Cooling_2nd_try\\September_2014\\091714\\67.98900K_500_2500_2.10000V_0.00000T_Sep17-2014__05-25-59_001_091714.bin", "mod time(min)"=58229845.983333334, "file format"=enum."binary", "power(V)"=2.1, "Magn Field(T) "=0.0}, {"temperature"=67.927, "temperature str"="67.92700", "file path"=path "D:/Data/Ultrasound/LSCO/LSCO22__130814c/5_Cooling_2nd_try/September_2014/091714/67.92700K_500_2500_2.10000V_0.00000T_Sep17-2014__05-27-18_001_091714.bin", "last mod"=timestamp(3493790838 s since 1904-01-01), "file name str"="D:\\Data\\Ultrasound\\LSCO\\LSCO22__130814c\\5_Cooling_2nd_try\\September_2014\\091714\\67.92700K_500_2500_2.10000V_0.00000T_Sep17-2014__05-27-18_001_091714.bin", "mod time(min)"=58229847.3, "file format"=enum."binary", "power(V)"=2.1, "Magn Field(T) "=0.0}, {"temperature"=67.865, "temperature str"="67.86500", "file path"=path "D:/Data/Ultrasound/LSCO/LSCO22__130814c/5_Cooling_2nd_try/September_2014/091714/67.86500K_500_2500_2.10000V_0.00000T_Sep17-2014__05-28-38_001_091714.bin", "last mod"=timestamp(3493790918 s since 1904-01-01), "file name str"="D:\\Data\\Ultrasound\\LSCO\\LSCO22__130814c\\5_Cooling_2nd_try\\September_2014\\091714\\67.86500K_500_2500_2.10000V_0.00000T_Sep17-2014__05-28-38_001_091714.bin", "mod time(min)"=58229848.63333333, "file format"=enum."binary", "power(V)"=2.1, "Magn Field(T) "=0.0}, {"temperature"=67.806, "temperature str"="67.80600", "file path"=path "D:/Data/Ultrasound/LSCO/LSCO22__130814c/5_Cooling_2nd_try/September_2014/091714/67.80600K_500_2500_2.10000V_0.00000T_Sep17-2014__05-29-57_001_091714.bin", "last mod"=timestamp(3493790997 s since 1904-01-01), "file name str"="D:\\Data\\Ultrasound\\LSCO\\LSCO22__130814c\\5_Cooling_2nd_try\\September_2014\\091714\\67.80600K_500_2500_2.10000V_0.00000T_Sep17-2014__05-29-57_001_091714.bin", "mod time(min)"=58229849.95, "file format"=enum."binary", "power(V)"=2.1, "Magn Field(T) "=0.0}, {"temperature"=67.745, "temperature str"="67.74500", "file path"=path "D:/Data/Ultrasound/LSCO/LSCO22__130814c/5_Cooling_2nd_try/September_2014/091714/67.74500K_500_2500_2.10000V_0.00000T_Sep17-2014__05-31-17_001_091714.bin", "last mod"=timestamp(3493791077 s since 1904-01-01), "file name str"="D:\\Data\\Ultrasound\\LSCO\\LSCO22__130814c\\5_Cooling_2nd_try\\September_2014\\091714\\67.74500K_500_2500_2.10000V_0.00000T_Sep17-2014__05-31-17_001_091714.bin", "mod time(min)"=58229851.28333333, "file format"=enum."binary", "power(V)"=2.1, "Magn Field(T) "=0.0}, {"temperature"=67.683, "temperature str"="67.68300", "file path"=path "D:/Data/Ultrasound/LSCO/LSCO22__130814c/5_Cooling_2nd_try/September_2014/091714/67.68300K_500_2500_2.10000V_0.00000T_Sep17-2014__05-32-36_001_091714.bin", "last mod"=timestamp(3493791156 s since 1904-01-01), "file name str"="D:\\Data\\Ultrasound\\LSCO\\LSCO22__130814c\\5_Cooling_2nd_try\\September_2014\\091714\\67.68300K_500_2500_2.10000V_0.00000T_Sep17-2014__05-32-36_001_091714.bin", "mod time(min)"=58229852.6, "file format"=enum."binary", "power(V)"=2.1, "Magn Field(T) "=0.0}, {"temperature"=67.625, "temperature str"="67.62500", "file path"=path "D:/Data/Ultrasound/LSCO/LSCO22__130814c/5_Cooling_2nd_try/September_2014/091714/67.62500K_500_2500_2.10000V_0.00000T_Sep17-2014__05-33-55_001_091714.bin", "last mod"=timestamp(3493791235 s since 1904-01-01), "file name str"="D:\\Data\\Ultrasound\\LSCO\\LSCO22__130814c\\5_Cooling_2nd_try\\September_2014\\091714\\67.62500K_500_2500_2.10000V_0.00000T_Sep17-2014__05-33-55_001_091714.bin", "mod time(min)"=58229853.916666664, "file 
